vi "Create Async FIFOs.vi"(8 "error in (no error)":errorcluster, 11 "State Vars":T1 {"CompiledSettings"."Result Ch Data Refs" format="%.0x"; "CompiledSettings"."Parameter Block Data Refs"."Data Reference" format="%.0x"}) -> (0 "error out":errorcluster, 3 "State Vars out":T1 {"CompiledSettings"."Result Ch Data Refs" format="%.0x"; "CompiledSettings"."Parameter Block Data Refs"."Data Reference" format="%.0x"})   [LabVIEW 2014, in "Waveform-Processing-Custom-Device Engine.lvlib"]
uses:
  Waveform-Processing-Custom-Device Engine.lvlib
  Types/Inline State Vars.ctl
  Types/Async FIFOs.ctl
  Shared/CompiledSettings.ctl
  <vilib>/NI Veristand/Custom Device API/Block Data Reference.ctl
  <vilib>/NI Veristand/Custom Device API/Data Reference.ctl
  <vilib>/NI Veristand/Custom Device API/Waveform Data Reference.ctl
  Shared/Waveform-Processing-Custom-Device Shared.lvlib
  <vilib>/NI Veristand/Custom Device API/Custom Device API.lvlib
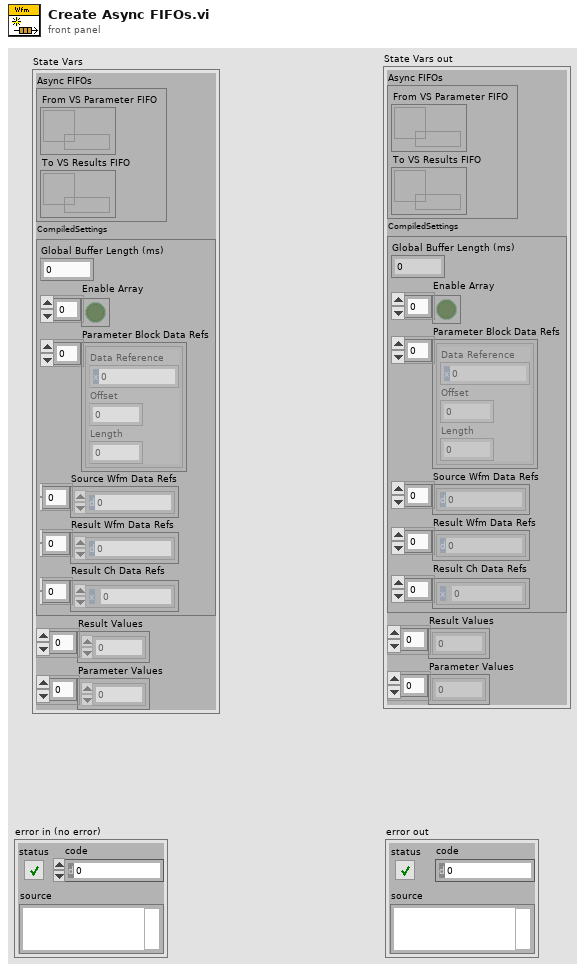
[diagram p1: front panel]
types:
  T1 = typedef "Waveform-Processing-Custom-Device Engine.lvlib/Inline State Vars.ctl" = cluster{"Async FIFOs":T2, "CompiledSettings":T3, "Result Values":dbl[], "Parameter Values":dbl[]}
  T2 = typedef "Waveform-Processing-Custom-Device Engine.lvlib/Async FIFOs.ctl" = cluster{"From VS Parameter FIFO":refnum<k33>, "To VS Results FIFO":refnum<k33>}
  T3 = typedef "Waveform-Processing-Custom-Device Shared.lvlib/CompiledSettings.ctl" = cluster{"Global Buffer Length (ms)":dbl, "Enable Array":bool[], "Parameter Block Data Refs":T4[], "Source Wfm Data Refs":T6[], "Result Wfm Data Refs":T6[], "Result Ch Data Refs":T5[]}
  T4 = typedef "Custom Device API.lvlib/Block Data Reference.ctl" = cluster{"Data Reference":T5, "Offset":i32, "Length":i32}
  T5 = typedef "Custom Device API.lvlib/Data Reference.ctl" = i32
  T6 = typedef "Custom Device API.lvlib/Waveform Data Reference.ctl" = i32
  T7 = cluster{"read mode":enum16{"polling", "blocking"}, "write mode":enum16{"polling", "blocking"}}
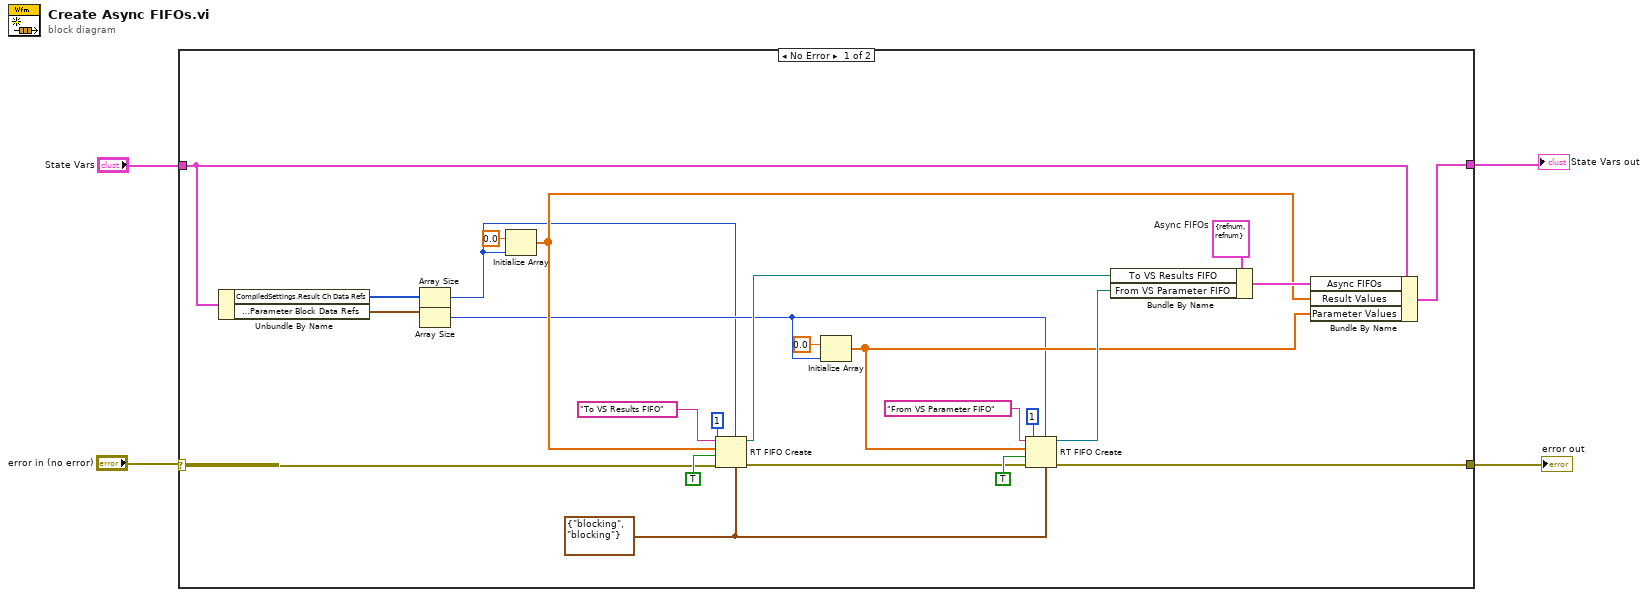
[diagram p0: block diagram]
diagram:
  n1 = case shown="No Error" "error in (no error)" {
    selector: "error in (no error)" -> [w16 w30]
    tunnel: [w28 w30] -> w4
    tunnel: "State Vars" -> [w14 w29]
    tunnel: [w12 w29] -> w1
    frame No Error {
      w27 = T7 {"read mode"=enum."blocking", "write mode"=enum."blocking"} ("r/w modes (polling,polling)")
      w22 = T2 {"From VS Parameter FIFO"=refnum, "To VS Results FIFO"=refnum}  # Async FIFOs
      n2 = Unbundle By Name(w14) -> ("CompiledSettings.Result Ch Data Refs"=w11:T5[], "CompiledSettings.Parameter Block Data Refs"=w15:T4[])
      n3 = Array Size(array=w11) -> (size(s)=w5:i32)
      n4 = Array Size(array=w15) -> (size(s)=w6:i32)
      n5 = Initialize Array(0.0, w5) -> (w8:dbl[])
      n6 = RT FIFO Create(0:"To VS Results FIFO" ("name (unnamed)"), 1:w8, 2:TRUE ("create if not found? (T)"), 3:w16, 4:u32 1 ("size (10)"), 6:w5, 7:w27) -> (8:w9:refnum<k33>, 11:w20:errorcluster)  [unwired: 1 in, 1 out]
      n7 = Initialize Array(0.0, w6) -> (w7:dbl[])
      n8 = RT FIFO Create(0:"From VS Parameter FIFO" ("name (unnamed)"), 1:w7, 2:TRUE ("create if not found? (T)"), 3:w20, 4:u32 1 ("size (10)"), 6:w6, 7:w27) -> (8:w25:refnum<k33>, 11:w28:errorcluster)  [unwired: 1 in, 1 out]
      n9 = Bundle By Name(cluster=w22, "To VS Results FIFO"=w9, "From VS Parameter FIFO"=w25) -> (w13:T2)
      n10 = Bundle By Name(cluster=w14, "Async FIFOs"=w13, "Result Values"=w8, "Parameter Values"=w7) -> (w12:T1)
    }
    frame Error {
    }
  }
  "error out" <- w4
  "State Vars out" <- w1
